vi "Set Tag Value.vi"(8 "error in (no error)":errorcluster, 9 "Tag Value":string, 10 "Tag Name":string, 11 "Input String":string) -> (0 "error out":errorcluster, 3 "Output String":string)   [LabVIEW 2016, in "SLL String.lvlib"]
doc: "Updates the tag value in the string for the provided tag name."
uses:
  SLL String.lvlib
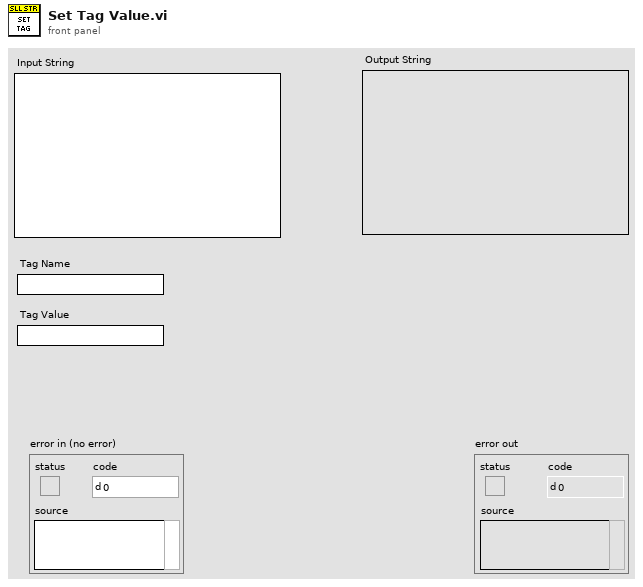
[diagram p1: front panel]
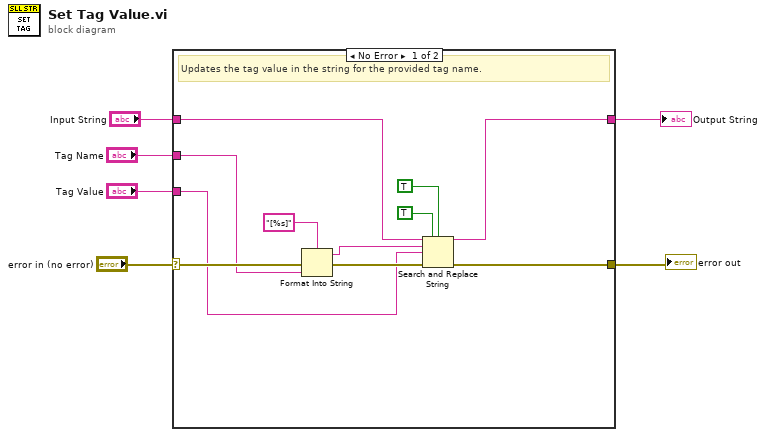
[diagram p0: block diagram]
diagram:
  n1 = case shown="No Error" "error in (no error)" {
    selector: "error in (no error)" -> [w17 w19]
    tunnel: "Input String" -> [w15 w18]
    tunnel: [w16 w19] -> w4
    tunnel: [w14 w18] -> w3
    tunnel: "Tag Name" -> [w9 _]
    tunnel: "Tag Value" -> [w7 _]
    frame No Error {
      # "Updates the tag value in the string for the provided tag name."
      n2 = Format Into String(format string="[%s]", error in=w17, w9) -> (resulting string=w8:string, error out=w11:errorcluster)  [unwired: 1 in]
      n3 = Search and Replace String(replace all?=TRUE ("replace all? (F)"), case sensitive?=TRUE ("ignore case? (F)"), input string=w15, search string=w8, replace string=w7, error in=w11) -> (result string=w14:string, error out=w16:errorcluster)  [unwired: 2 in, 2 out]
    }
    frame Error {
    }
  }
  "error out" <- w4
  "Output String" <- w3
